vi "GUI RGB.vi"(9 "Blue":u8, 10 "Green":u8, 11 "Red":u8) -> (3 "result":u32)   [LabVIEW 2011, in "User Interface VIs.lvlib"]
uses:
  User Interface VIs.lvlib
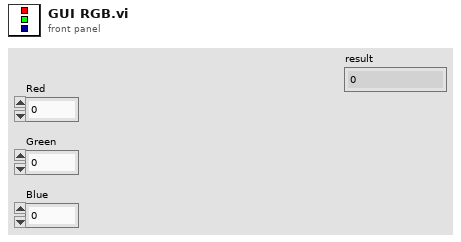
[diagram p1: front panel]
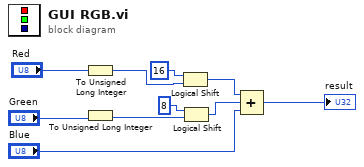
[diagram p0: block diagram]
diagram:
  n1 = To Unsigned Long Integer(number="Red") -> (unsigned 32bit integer=w3:u32)
  n2 = To Unsigned Long Integer(number="Green") -> (unsigned 32bit integer=w1:u32)
  n3 = Logical Shift(y=16 ("x"), x=w3) -> (x << y=w6:u32)
  n4 = Logical Shift(y=8 ("x"), x=w1) -> (x << y=w7:u32)
  n5 = Compound Arithmetic op=ADD(w6, w7, "Blue") -> (→"result":u32)
